vi "Read Info from File.vi"(8 "error in (no error)":errorcluster, 11 "LabVIEW Project File in":refnum<class "LabVIEW Project File.lvclass">) -> (0 "error out":errorcluster, 3 "LabVIEW Project File out":refnum<class "LabVIEW Project File.lvclass">)   [LabVIEW 2020, in "Save for Previous Version.lvlib" / "LabVIEW Project File.lvclass"]
uses:
  LabVIEW Project File.lvclass
  \\Mac\Home/JKI/GitHub/save-for-previous-labview-version/source/File/File.lvclass/File.lvclass
  \\Mac\Home/JKI/GitHub/save-for-previous-labview-version/source/LabVIEW File/LabVIEW File.lvclass
  File/File.lvclass/File.lvclass/File.ctl
  LabVIEW File/LabVIEW File.lvclass/LabVIEW File.ctl
  File/File.lvclass/Read Path.vi
  LabVIEW File/Write Version String.vi
  LabVIEW File/Write Version Number.vi
  LabVIEW File/LabVIEW File.lvclass
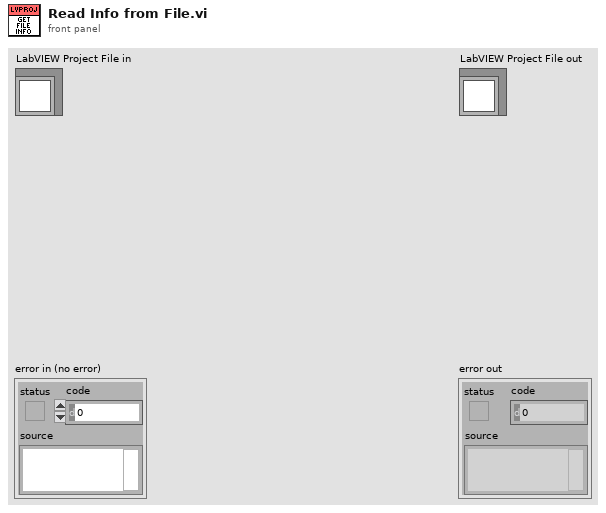
[diagram p1: front panel]
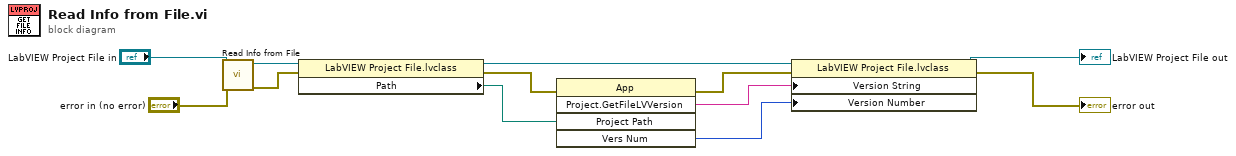
[diagram p0: block diagram]
diagram:
  n1 = call-parent "Read Info from File.vi"("error in (no error)"="error in (no error)", "LabVIEW File in"="LabVIEW Project File in") -> ("error out"=w8:errorcluster, "LabVIEW File out"=w10:refnum<class "LabVIEW Project File.lvclass">)  [unwired: 8 in]
  n2 = property class="LabVIEW Project File.lvclass"(reference=w10, error in=w8) -> (reference out=w9:refnum<class "LabVIEW Project File.lvclass">, error out=w6:errorcluster, "Path"=w7:path)
  n3 = invoke class="App" method="Project.GetFileLVVersion"(error in=w6, "Project Path"=w7) -> (error out=w5:errorcluster, "Project.GetFileLVVersion"=w12:string, "Vers Num"=w11:u32)  [unwired: 3 in, 2 out]
  n4 = property class="LabVIEW Project File.lvclass"(reference=w9, error in=w5, "Version String"=w12, "Version Number"=w11) -> (reference out=→"LabVIEW Project File out":refnum<class "LabVIEW Project File.lvclass">, error out=→"error out":errorcluster)
